vi "Plotter stop FGV.vi"(8 "error in":errorcluster, 10 "Stop in":bool, 11 "Function":enum16{"Read", "Write", "Clear"}(ring)) -> (0 "error out":errorcluster, 3 "Stop out":bool)   [LabVIEW 2020]
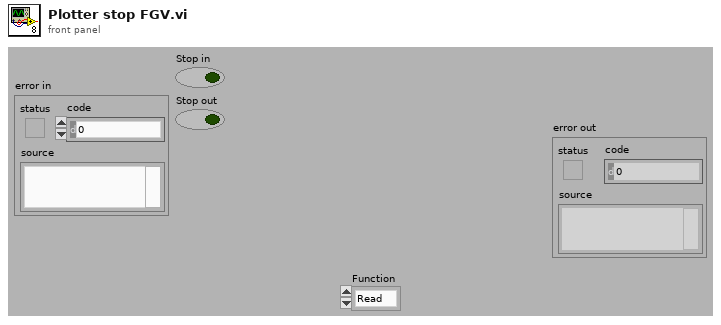
[diagram p1: front panel]
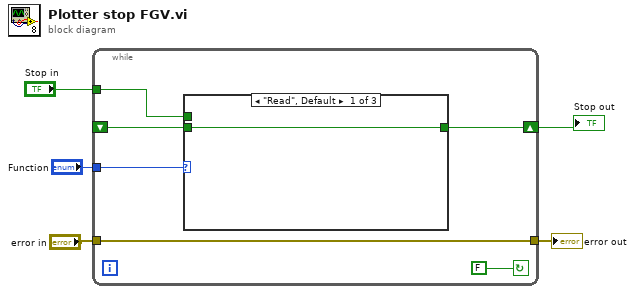
[diagram p0: block diagram]
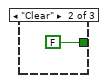
[diagram p2: hidden frame]
diagram:
  n1 = while {
    shift-right: [w9] -> w1
    shift-left: _ -> [w8]
    tunnel: "Function" -> [w11]
    tunnel: "Stop in" -> [w10]
    tunnel: "error in" -> [w6]
    tunnel: [w6] -> w3
    stop <- FALSE continue-if-true
    n2 = case shown="\"Read\", Default" w11 {
      tunnel: w10 -> [_ _ w14]
      tunnel: [w12 FALSE ("Stop") w14] -> w9
      tunnel: w8 -> [w12 _ _]
      frame "Read", Default {
      }
      frame "Clear" {
      }
      frame "Write" {
      }
    }
  }
  "error out" <- w3
  "Stop out" <- w1
